vi "UTIL Butterworth Process.vi"(4 "Bandstop?":bool, 6 "Testing":bool, 7 "Filter Order":i32=3, 8 "Error In":errorcluster, 9 "Continue":bool, 10 "Filter Freqs":T1, 11 "Signal In":waveform(dbl)) -> (0 "Error Out":errorcluster, 2 "Power":dbl, 3 "Filtered Signal Out":waveform(dbl))   [LabVIEW 2010]
doc: "This processes signals using a 3rd order Butterworth Filter, whose type (Low Pass, High Pass, BandPass) are determined by the presence or absence of non-zero High Cut and Low Cut Filter Frequencies. Note that the LabVIEW Butterworth Filter is not entirely \"logical\" -- you wire to the Low Cut input for both High Pass and Low Pass. If no Filter Frequencies are specified, the default Low Pass filter will be used.\n\nThe filterred data are returned, along with the log of the mean, squared (log Power).\n\nA Testing input (default False), if True, replaces the Filter with a \"DC\" filter, namely the constant mean value of the waveform.\n\nInputs:\n Signal In Waveform\n\n Filter Freqs Cluster of Dbl, High Cut, Low Cut\n Continue Boolean, set True if this a continuation of an on-going Waveform\n Error In\nOutputs:\n Filtered Signal Out Waveform\n Power Log of mean square Filtered Signal\n Error Out"
uses:
  Types/TYPE Filter Freqs.ctl
  <vilib>/Analysis/3filter.llb/Butterworth Filter (DBL).vi
  <vilib>/Analysis/NI_AALBase.lvlib
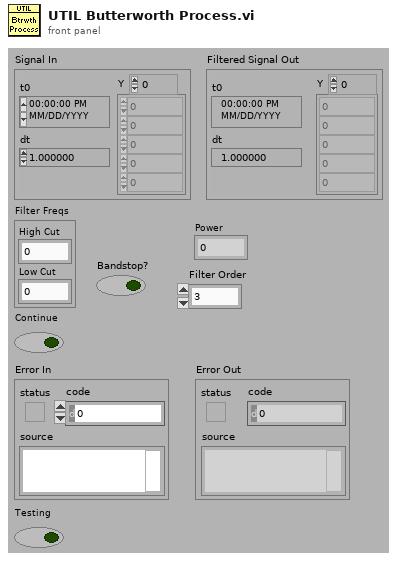
[diagram p1: front panel]
types:
  T1 = typedef "TYPE Filter Freqs.ctl" = cluster{"High Cut":dbl, "Low Cut":dbl}
  T2 = typedef "NI_AALBase.lvlib/Filter Passband Type.ctl" = enum32{"Lowpass", "Highpass", "Bandpass", "Bandstop"}
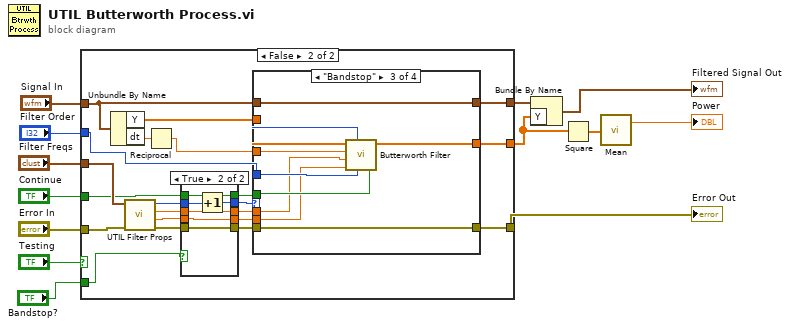
[diagram p0: block diagram]
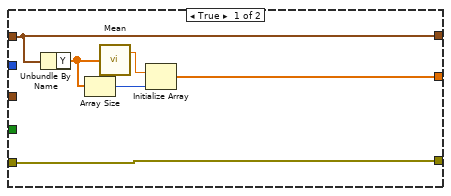
[diagram p2: hidden frame]
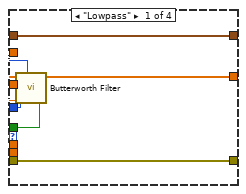
[diagram p4: hidden frame]
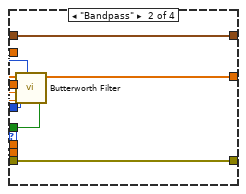
[diagram p5: hidden frame]
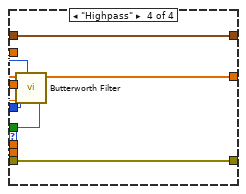
[diagram p6: hidden frame]
diagram:
  n1 = case shown="False" "Testing" {
    tunnel: "Error In" -> [w19 w40]
    tunnel: "Filter Freqs" -> [_ w39]
    tunnel: [w19 w38] -> w11
    tunnel: "Signal In" -> [w18 w37]
    tunnel: "Continue" -> [_ w22]
    tunnel: [w18 w35] -> w7
    tunnel: [w16 w34] -> w6
    tunnel: "Filter Order" -> [_ w31]
    tunnel: "Bandstop?" -> [_ w30]
    frame True {
      n2 = Unbundle By Name(w18) -> ("Y"=w15:dbl[])
      n3 = Array Size(array=w15) -> (size(s)=w14:i32)
      n4 = call <vilib>:"Mean.vi"("X"=w15) -> ("mean"=w17:dbl)  [unwired: 1 out]
      n5 = Initialize Array(w17, w14) -> (w16:dbl[])
    }
    frame False {
      n6 = Unbundle By Name(w37) -> ("Y"=w36:dbl[], "dt"=w33:dbl)
      n7 = call "UTIL Filter Props.vi"("Error In"=w40, "Filter Freqs"=w39) -> ("Error Out"=w29:errorcluster, "Low Cut"=w27:dbl, "High Cut"=w25:dbl, "Filter Type"=w23:T2)  [unwired: 6 in]
      n8 = Reciprocal(x=w33) -> (1/x=w32:dbl)
      n9 = case shown="True" w30 {
        tunnel: w29 -> [w41 w51]
        tunnel: [w41 w51] -> w28
        tunnel: [w42 w50] -> w26
        tunnel: w27 -> [w42 w50]
        tunnel: w25 -> [w43 w49]
        tunnel: [w43 w49] -> w24
        tunnel: w23 -> [w44 w47]
        tunnel: w22 -> [w45 w48]
        tunnel: [w45 w48] -> w21
        tunnel: [w44 w46] -> w20
        frame False {
        }
        frame True {
          n10 = Increment(x=w47) -> (x+1=w46:T2)
        }
      }
      n11 = case shown="\"Bandstop\"" w20 {
        selector: w20 -> [w54 w68 w74 w87]
        tunnel: w28 -> [w58 w66 w79 w86]
        tunnel: [w58 w66 w79 w86] -> w38
        tunnel: w24 -> [w53 w63 w72 _]
        tunnel: w26 -> [_ w67 w71 w82]
        tunnel: w37 -> [w56 w64 w77 w84]
        tunnel: w36 -> [w55 w62 w76 w83]
        tunnel: w32 -> [w59 w69 w80 w88]
        tunnel: [w57 w65 w78 w85] -> w34
        tunnel: [w56 w64 w77 w84] -> w35
        tunnel: w21 -> [w60 w70 w75 w89]
        tunnel: w31 -> [w52 w61 w73 w81]
        frame "Lowpass" {
          n12 = call-poly <vilib>:"Butterworth Filter.vi"("init/cont (init:F)"=w60, "order"=w52, "filter type"=w54, "low cutoff freq: fl"=w53, "sampling freq: fs"=w59, "X"=w55) -> ("Filtered X"=w57:dbl[])  [unwired: 2 in, 1 out]
        }
        frame "Bandpass" {
          n13 = call-poly <vilib>:"Butterworth Filter.vi"("init/cont (init:F)"=w70, "order"=w61, "filter type"=w68, "low cutoff freq: fl"=w67, "high cutoff freq: fh"=w63, "sampling freq: fs"=w69, "X"=w62) -> ("Filtered X"=w65:dbl[])  [unwired: 1 in, 1 out]
        }
        frame "Bandstop" {
          n14 = call-poly <vilib>:"Butterworth Filter.vi"("init/cont (init:F)"=w75, "order"=w73, "filter type"=w74, "low cutoff freq: fl"=w71, "high cutoff freq: fh"=w72, "sampling freq: fs"=w80, "X"=w76) -> ("Filtered X"=w78:dbl[])  [unwired: 1 in, 1 out]
        }
        frame "Highpass" {
          n15 = call-poly <vilib>:"Butterworth Filter.vi"("init/cont (init:F)"=w89, "order"=w81, "filter type"=w87, "low cutoff freq: fl"=w82, "sampling freq: fs"=w88, "X"=w83) -> ("Filtered X"=w85:dbl[])  [unwired: 2 in, 1 out]
        }
      }
    }
  }
  "Error Out" <- w11
  n16 = Bundle By Name(cluster=w7, "Y"=w6) -> (→"Filtered Signal Out":waveform(dbl))
  n17 = Square(x=w6) -> (x^2=w5:dbl[])
  n18 = call <vilib>:"Mean.vi"("X"=w5) -> ("mean"=→"Power":dbl)  [unwired: 1 out]
